vi "ThreadPlot.vi"(7 "数据通知器":refnum<notifier>, 8 "error in (no error)":errorcluster caption="错误输入（无错误）", 10 "传感器显示UI控件":T1, 11 "Message Queues":T2 caption="消息队列") -> (0 "error out":errorcluster caption="错误输出")   [LabVIEW 2015]
uses:
  support/Message Queue/All Message Queues.ctl
  support/Message Queue/Message Cluster.ctl
  controls/ValueUI Data.ctl
  Measure Type.ctl
  <vilib>/Utility/error.llb/Error Cluster From Error Code.vi
  support/Message Queue/Enqueue Message (Single).vi
  <vilib>/ErrorRing/Error Ring.xnode
  support/Message Queue/Message Queue.lvlib
  Acquisition/Acquisition.lvlib
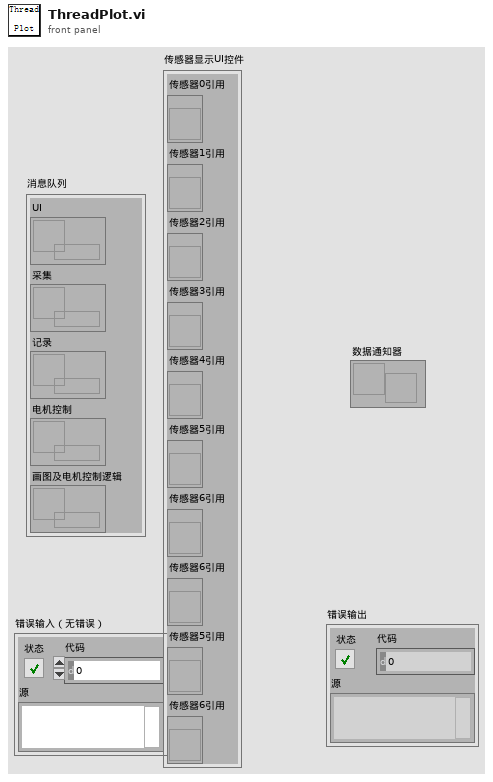
[diagram p1: front panel]
types:
  T1 = typedef "ValueUI Data.ctl" = cluster{"数据1引用":refnum<vi>, "数据2引用":refnum<vi>, "数据3引用":refnum<vi>, "传感器0引用":refnum<vi>, "传感器1引用":refnum<vi>, "传感器2引用":refnum<vi>, "传感器3引用":refnum<vi>, "传感器4引用":refnum<vi>, "传感器5引用":refnum<vi>, "传感器6引用":refnum<vi>}
  T2 = typedef "Message Queue.lvlib/All Message Queues.ctl" = cluster{"UI":refnum<queue>, "Acquisition":refnum<queue>, "Logging":refnum<queue>, "plot logic":refnum<queue>, "Action Control":refnum<queue>}
  T3 = typedef "Measure Type.ctl" = enum16{"啮合", "退回", "功能", "力特性", "内泄漏", "分中", "对中"}
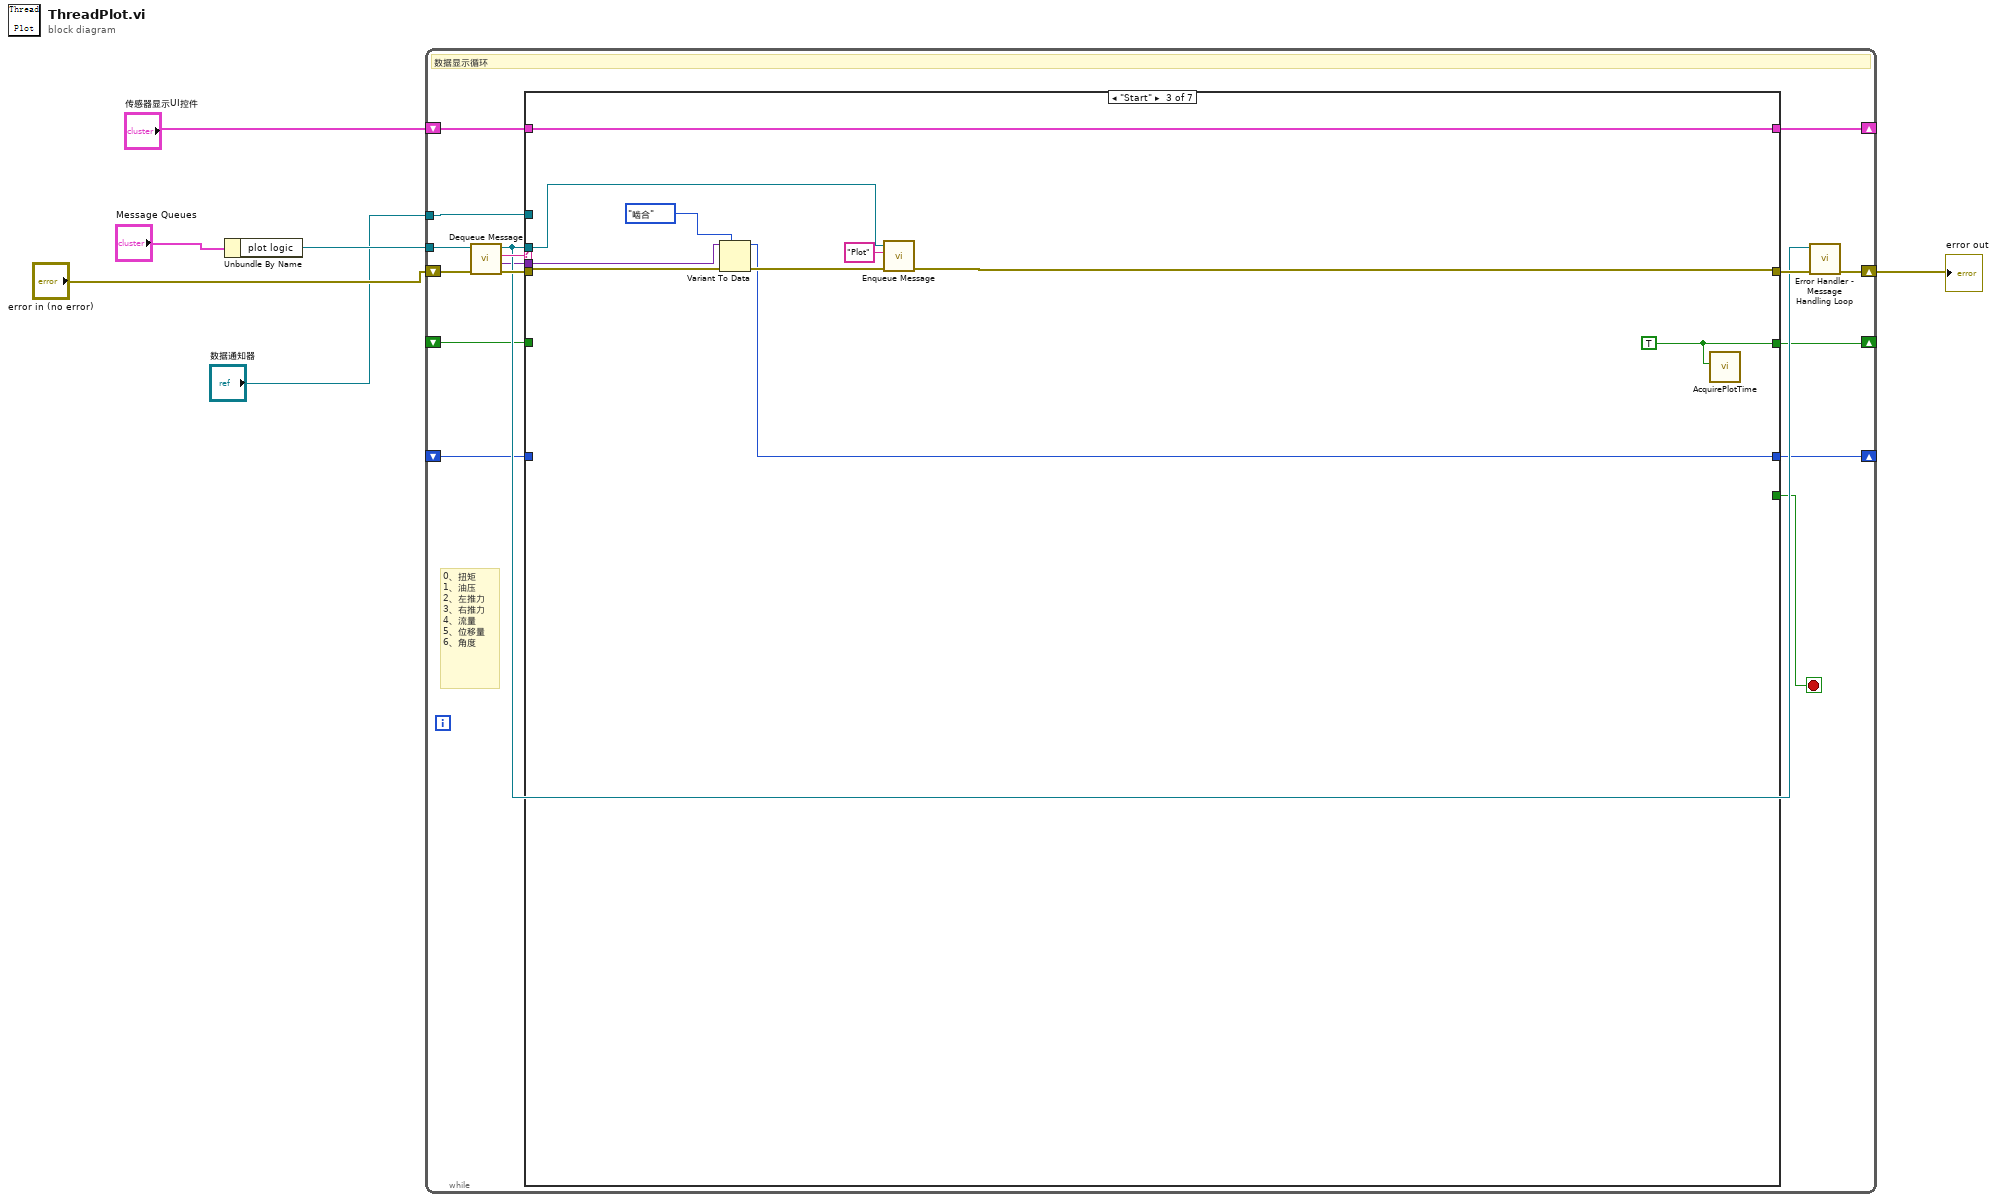
[diagram p0: block diagram]
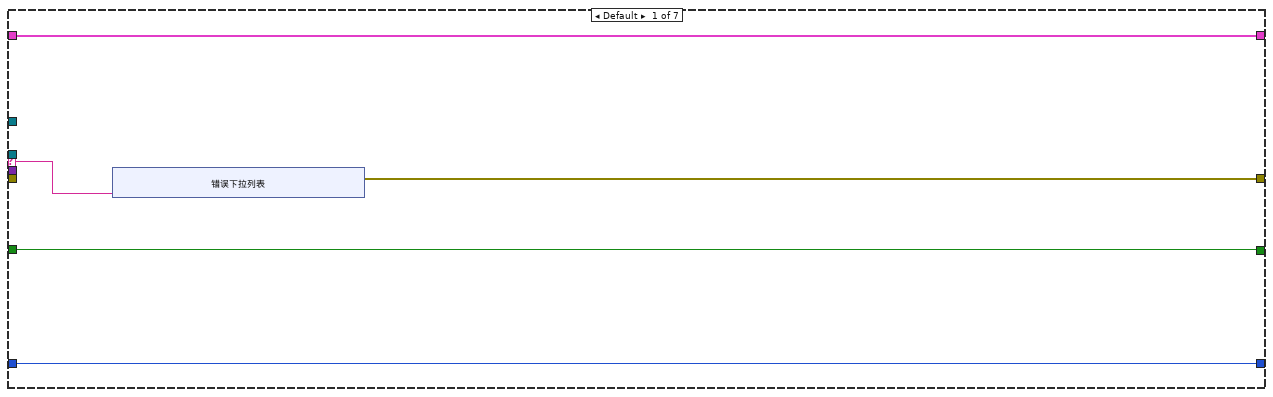
[diagram p2: hidden frame]
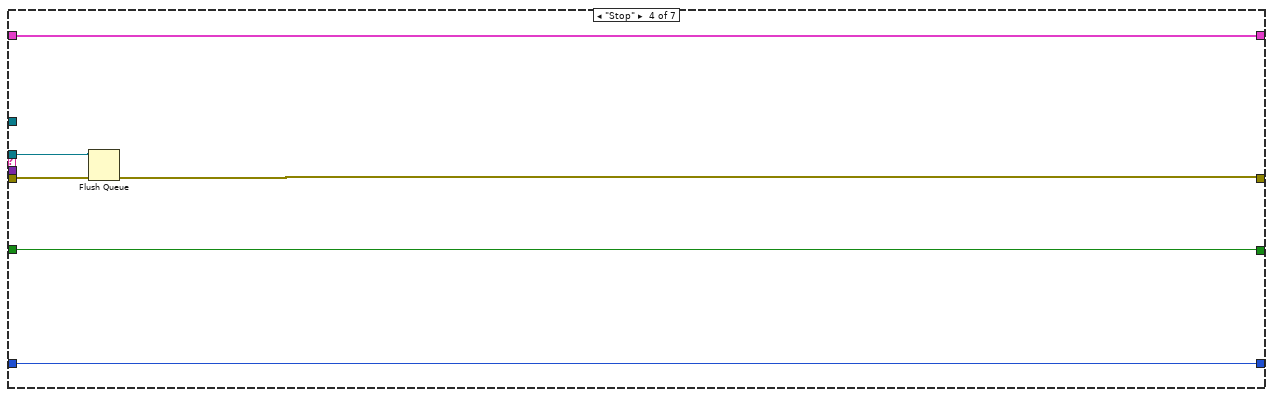
[diagram p4: hidden frame]
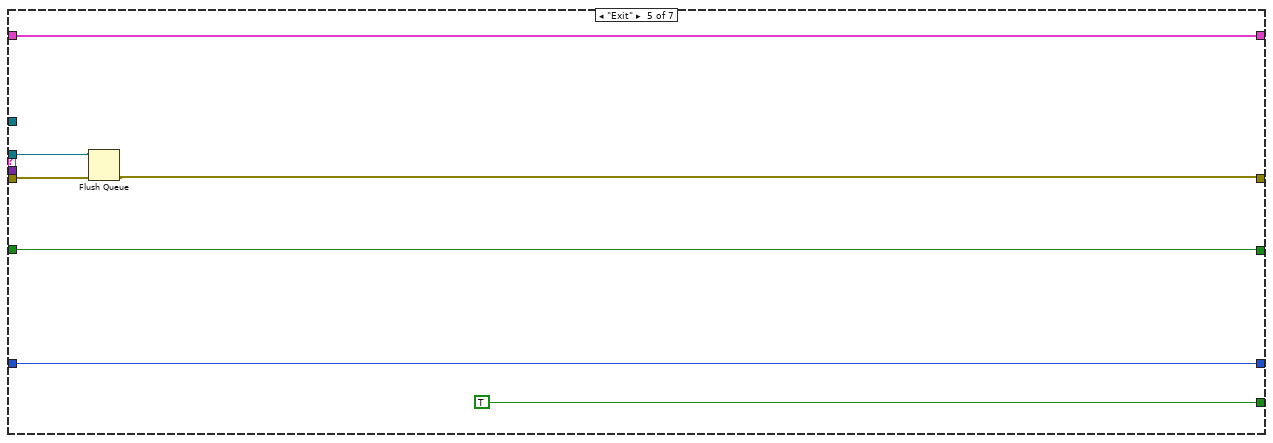
[diagram p5: hidden frame]
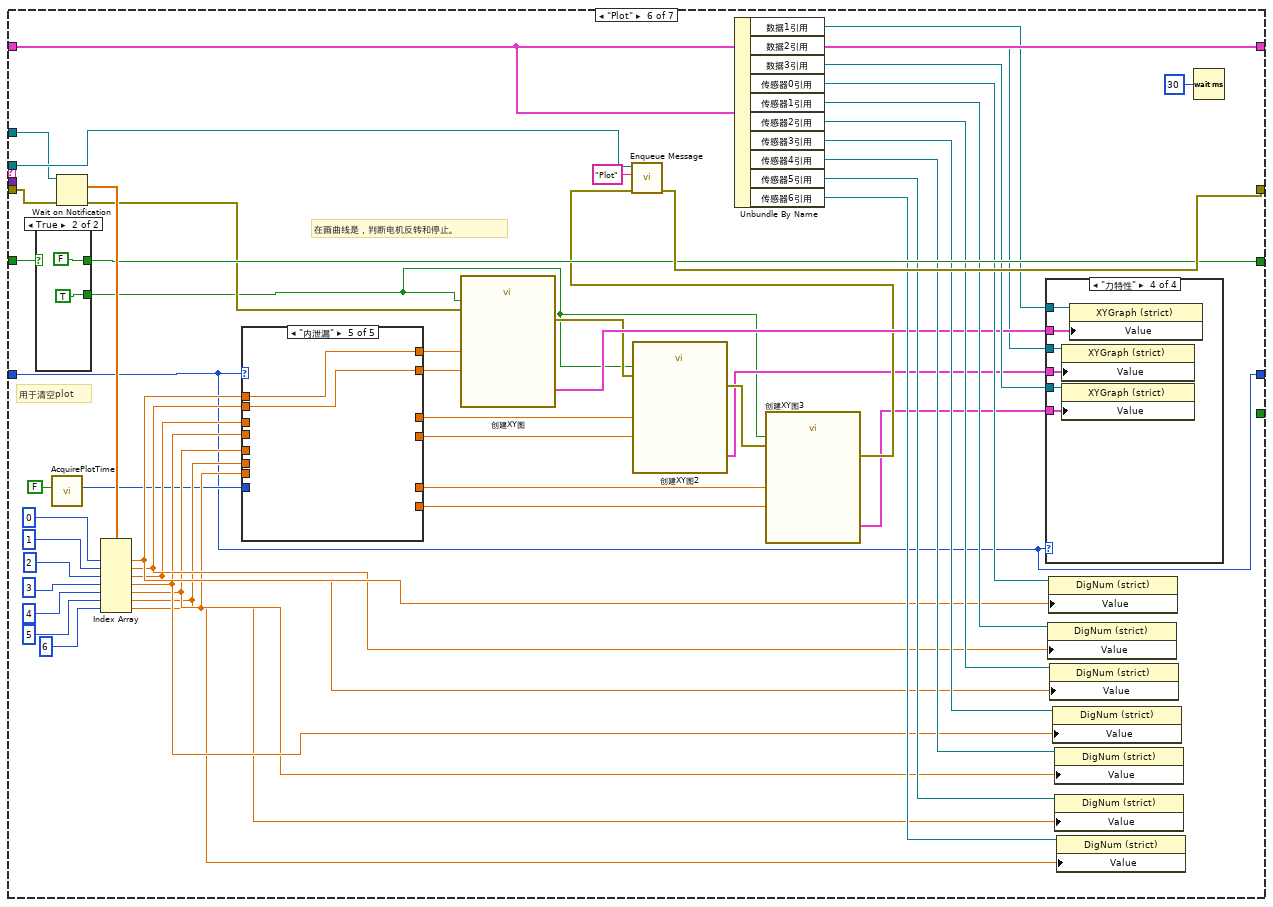
[diagram p6: hidden frame]
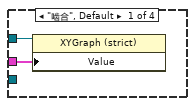
[diagram p7: hidden frame]
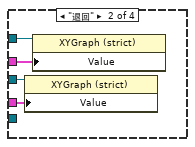
[diagram p8: hidden frame]
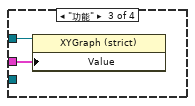
[diagram p9: hidden frame]
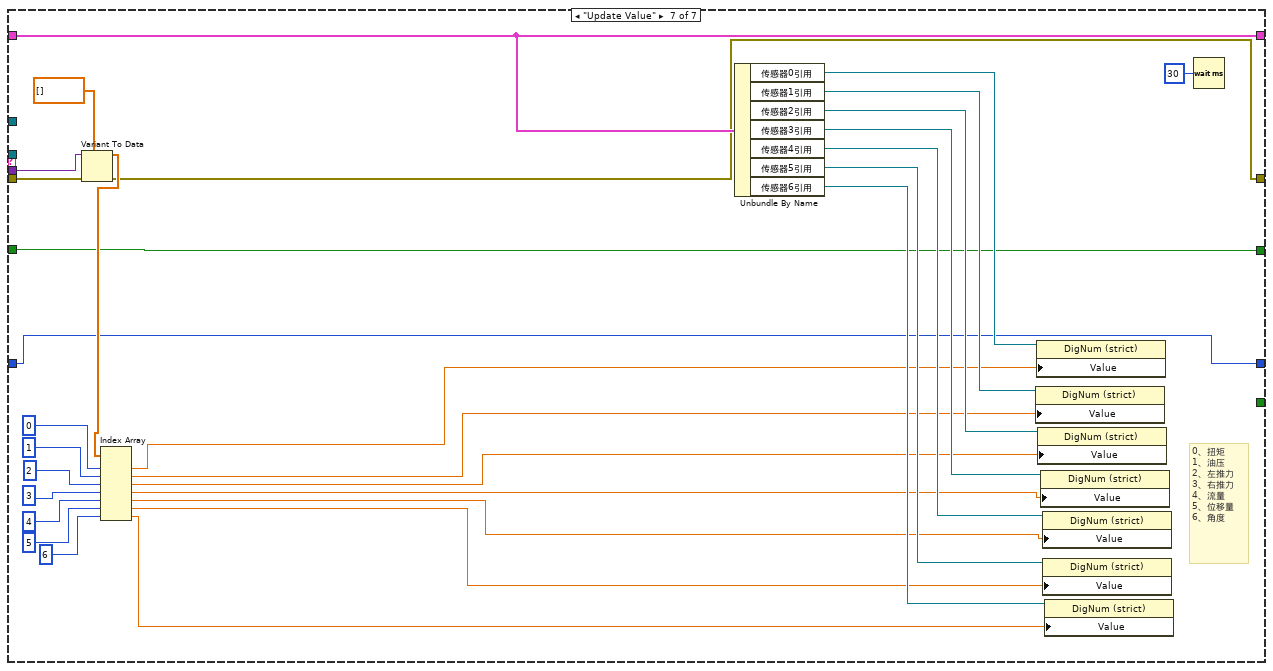
[diagram p15: hidden frame]
diagram:
  n1 = Unbundle By Name("Message Queues") -> ("plot logic"=w6:refnum<queue>)
  n2 = while "Data Display Loop" {
    tunnel: "数据通知器" -> [w15]
    tunnel: w6 -> [w22]
    shift-right: [w17] -> w1
    shift-left: "error in (no error)" -> [w21]
    shift-right: [w12] -> _
    shift-left: _ -> [w11]
    shift-right: [w9] -> _
    shift-left: "传感器显示UI控件" -> [w10]
    shift-right: [w7] -> _
    shift-left: _ -> [w8]
    stop <- w14 stop-if-true
    # "0、扭矩\n1、油压\n2、左推力\n3、右推力\n4、流量\n5、位移量\n6、角度"
    # "数据显示循环"
    n3 = call "Dequeue Message.vi"("error in (no error)"=w21, "Message Queue"=w22) -> ("error out"=w19:errorcluster, "Message Data"=w13:variant, "Message"=w18:string, "dup Message Queue"=w16:refnum<queue>)  [unwired: 6 in]
    n4 = case shown="\"Start\"" w18 {
      selector: w18 -> [w26 _ _ _ _ _ _]
      tunnel: [w27 w38 w46 w53 w59 w101 w142] -> w20
      tunnel: w19 -> [_ w38 w43 w54 w61 w109 w147]
      tunnel: w16 -> [_ _ w48 w52 w60 w112 _]
      tunnel: w15 -> [_ _ _ _ _ w110 _]
      tunnel: [_ _ _ _ TRUE _ _] -> w14
      tunnel: w13 -> [_ _ w41 _ _ _ w146]
      tunnel: [w25 w37 w44 w51 w57 w97 w143] -> w12
      tunnel: w11 -> [w25 w37 _ w51 w57 w98 w143]
      tunnel: w10 -> [w24 w36 w45 w50 w56 w96 w162]
      tunnel: [w24 w36 w45 w50 w56 w96 w162] -> w9
      tunnel: w8 -> [w23 w35 _ w49 w55 w62 w141]
      tunnel: [w23 w35 w39 w49 w55 w62 w141] -> w7
      frame Default {
        n5 = xnode "错误下拉列表"("parameter 0"=w26) -> ("error out"=w27:errorcluster)
      }
      frame "Initialize" {
      }
      frame "Start" {
        w44 = TRUE
        n6 = Variant To Data(error in=w43, type=Measure_Type."啮合" ("画曲线类型"), Variant=w41) -> (data=w39:T3, error out=w42:errorcluster)
        n7 = call-poly "Enqueue Message.vi"("error in (no error)"=w42, "Message"="Plot", "Message Queue"=w48) -> ("error out"=w46:errorcluster)  [unwired: 7 in, 1 out]
        n8 = call "AcquirePlotTime.vi"("重启？"=w44) -> ()  [unwired: 10 in, 1 out]
      }
      frame "Stop" {
        n9 = Flush Queue(queue=w52, error in (no error)=w54) -> (error out=w53:errorcluster)  [unwired: 2 out]
      }
      frame "Exit" {
        n10 = Flush Queue(queue=w60, error in (no error)=w61) -> (error out=w59:errorcluster)  [unwired: 2 out]
      }
      frame "Plot" {
        # "用于清空plot"
        # "在画曲线是，判断电机反转和停止。"
        n11 = case shown="True" w98 {
          tunnel: [_ TRUE] -> w63
          tunnel: [_ FALSE] -> w97
          frame False {
          }
          frame True {
          }
        }
        n12 = call "AcquirePlotTime.vi"("重启？"=FALSE) -> ("时间"=w71:u32)  [unwired: 10 in]
        n13 = Wait on Notification(notifier=w110, error in (no error)=w109) -> (notification=w100:dbl[], error out=w64:errorcluster)  [unwired: 2 in, 2 out]
        n14 = Index Array(array=w100, index #1=0 ("索引"), index #2=1 ("索引"), index #3=2 ("索引"), index #4=3 ("索引"), index #5=4 ("索引"), index #6=5 ("索引"), index #7=6 ("索引")) -> (element #1=w81:dbl, element #2=w80:dbl, element #3=w79:dbl, element #4=w78:dbl, element #5=w77:dbl, element #6=w76:dbl, element #7=w75:dbl)
        n15 = case shown="\"内泄漏\"" w62 {
          tunnel: w81 -> [w127 _ w132 w134 w138]
          tunnel: w80 -> [_ _ _ w136 w137]
          tunnel: w79 -> [_ w130 _ _ _]
          tunnel: w78 -> [_ w129 _ _ _]
          tunnel: w77 -> [_ _ _ _ _]
          tunnel: w76 -> [_ _ _ _ _]
          tunnel: w75 -> [w128 _ w133 w135 _]
          tunnel: [w128 w131 w133 w134 w138] -> w74
          tunnel: [w127 w130 w132 w136 w137] -> w73
          tunnel: w71 -> [_ w131 _ _ _]
          tunnel: [_ w131 _ w135 _] -> w70
          tunnel: [_ w129 _ w136 _] -> w69
          tunnel: [_ _ _ w135 _] -> w68
          tunnel: [_ _ _ w134 _] -> w67
          frame "啮合", Default {
          }
          frame "退回" {
          }
          frame "功能" {
          }
          frame "力特性" {
          }
          frame "内泄漏" {
          }
        }
        n16 = call "创建XY图"("error in (no error)"=w64, "Reset"=w63, "Y Input"=w73, "X Input"=w74) -> ("error out"=w84:errorcluster, "XY Graph"=w87:cluster{"X":dbl[], "Y":dbl[]}[])  [unwired: 6 in]
        n17 = call "创建XY图2"("error in (no error)"=w84, "Reset"=w63, "Y Input"=w69, "X Input"=w70) -> ("error out"=w83:errorcluster, "XY Graph"=w66:cluster{"X":dbl[], "Y":dbl[]}[])  [unwired: 6 in]
        n18 = Unbundle By Name(w96) -> ("数据1引用"=w85:refnum<vi>, "数据2引用"=w86:refnum<vi>, "数据3引用"=w95:refnum<vi>, "传感器0引用"=w94:refnum<vi>, "传感器1引用"=w93:refnum<vi>, "传感器2引用"=w92:refnum<vi>, "传感器3引用"=w91:refnum<vi>, "传感器4引用"=w90:refnum<vi>, "传感器5引用"=w89:refnum<vi>, "传感器6引用"=w88:refnum<vi>)
        n19 = call "创建XY图3"("error in (no error)"=w83, "Reset"=w63, "Y Input"=w67, "X Input"=w68) -> ("error out"=w82:errorcluster, "XY Graph"=w65:cluster{"X":dbl[], "Y":dbl[]}[])  [unwired: 6 in]
        n20 = call-poly "Enqueue Message.vi"("error in (no error)"=w82, "Message"="Plot", "Message Queue"=w112) -> ("error out"=w101:errorcluster)  [unwired: 7 in, 1 out]
        n21 = case shown="\"力特性\"" w62 {
          tunnel: w95 -> [_ _ _ w126]
          tunnel: w87 -> [w114 w118 w120 w125]
          tunnel: w86 -> [_ w117 _ w124]
          tunnel: w85 -> [w113 w116 w119 w123]
          tunnel: w66 -> [_ w115 _ w122]
          tunnel: w65 -> [_ _ _ w121]
          frame "啮合", Default {
            n22 = property class="XYGraph (strict)"(reference=w113, "Value"=w114) -> ()  [unwired: 1 in, 2 out]
          }
          frame "退回" {
            n23 = property class="XYGraph (strict)"(reference=w117, "Value"=w115) -> ()  [unwired: 1 in, 2 out]
            n24 = property class="XYGraph (strict)"(reference=w116, "Value"=w118) -> ()  [unwired: 1 in, 2 out]
          }
          frame "功能" {
            n25 = property class="XYGraph (strict)"(reference=w119, "Value"=w120) -> ()  [unwired: 1 in, 2 out]
          }
          frame "力特性" {
            n26 = property class="XYGraph (strict)"(reference=w124, "Value"=w122) -> ()  [unwired: 1 in, 2 out]
            n27 = property class="XYGraph (strict)"(reference=w126, "Value"=w121) -> ()  [unwired: 1 in, 2 out]
            n28 = property class="XYGraph (strict)"(reference=w123, "Value"=w125) -> ()  [unwired: 1 in, 2 out]
          }
        }
        n29 = property class="DigNum (strict)"(reference=w93, "Value"=w80) -> ()  [unwired: 1 in, 2 out]
        n30 = property class="DigNum (strict)"(reference=w94, "Value"=w81) -> ()  [unwired: 1 in, 2 out]
        n31 = property class="DigNum (strict)"(reference=w92, "Value"=w79) -> ()  [unwired: 1 in, 2 out]
        n32 = property class="DigNum (strict)"(reference=w91, "Value"=w78) -> ()  [unwired: 1 in, 2 out]
        n33 = property class="DigNum (strict)"(reference=w90, "Value"=w77) -> ()  [unwired: 1 in, 2 out]
        n34 = property class="DigNum (strict)"(reference=w89, "Value"=w76) -> ()  [unwired: 1 in, 2 out]
        n35 = property class="DigNum (strict)"(reference=w88, "Value"=w75) -> ()  [unwired: 1 in, 2 out]
        n36 = Wait (ms)(milliseconds to wait=u32 30 ("等待时间（毫秒）")) -> ()  [unwired: 1 out]
      }
      frame "Update Value" {
        # "0、扭矩\n1、油压\n2、左推力\n3、右推力\n4、流量\n5、位移量\n6、角度"
        n37 = Variant To Data(error in=w147, type=dbl[] [], Variant=w146) -> (data=w144:dbl[], error out=w142:errorcluster)
        n38 = Index Array(array=w144, index #1=0 ("索引"), index #2=1 ("索引"), index #3=2 ("索引"), index #4=3 ("索引"), index #5=4 ("索引"), index #6=5 ("索引"), index #7=6 ("索引")) -> (element #1=w154:dbl, element #2=w153:dbl, element #3=w152:dbl, element #4=w151:dbl, element #5=w150:dbl, element #6=w149:dbl, element #7=w148:dbl)
        n39 = Unbundle By Name(w162) -> ("传感器0引用"=w161:refnum<vi>, "传感器1引用"=w160:refnum<vi>, "传感器2引用"=w159:refnum<vi>, "传感器3引用"=w158:refnum<vi>, "传感器4引用"=w157:refnum<vi>, "传感器5引用"=w156:refnum<vi>, "传感器6引用"=w155:refnum<vi>)
        n40 = property class="DigNum (strict)"(reference=w160, "Value"=w153) -> ()  [unwired: 1 in, 2 out]
        n41 = property class="DigNum (strict)"(reference=w161, "Value"=w154) -> ()  [unwired: 1 in, 2 out]
        n42 = property class="DigNum (strict)"(reference=w159, "Value"=w152) -> ()  [unwired: 1 in, 2 out]
        n43 = property class="DigNum (strict)"(reference=w158, "Value"=w151) -> ()  [unwired: 1 in, 2 out]
        n44 = property class="DigNum (strict)"(reference=w157, "Value"=w150) -> ()  [unwired: 1 in, 2 out]
        n45 = property class="DigNum (strict)"(reference=w156, "Value"=w149) -> ()  [unwired: 1 in, 2 out]
        n46 = property class="DigNum (strict)"(reference=w155, "Value"=w148) -> ()  [unwired: 1 in, 2 out]
        n47 = Wait (ms)(milliseconds to wait=u32 30 ("等待时间（毫秒）")) -> ()  [unwired: 1 out]
      }
    }
    n48 = call "Error Handler - Message Handling Loop.vi"("error in (no error)"=w20, "Message Queue"=w16) -> ("dup error in"=w17:errorcluster)  [unwired: 8 in, 1 out]
  }
  "error out" <- w1
